vi "Invert_Digital_Data.vi"(8 "error in (no error)":errorcluster, 10 "Index to invert":i32=3, 11 "DO WF":digitalwaveform[](graph)=[{"t0"=timestamp(0 s since 1904-01-01), "dt"=0.0001, "Y"={"transitions"=[], "data"=array90000x1[90000 elements]}}, {"t0"=timestamp(0 s since 1904-01-01), "dt"=0.0001, "Y"={"transitions"=[], "data"=array90000x1[90000 elements]}}, {"t0"=timestamp(0 s since 1904-01-01), "dt"=0.0001, "Y"={"transitions"=[], "data"=array90000x1[90000 elements]}}]) -> (0 "error out":errorcluster, 3 "DO WF 2":digitalwaveform[](graph)=[{"t0"=timestamp(0 s since 1904-01-01), "dt"=0.0001, "Y"={"transitions"=[], "data"=array90000x1[90000 elements]}}, {"t0"=timestamp(0 s since 1904-01-01), "dt"=0.0001, "Y"={"transitions"=[], "data"=array90000x1[90000 elements]}}, {"t0"=timestamp(0 s since 1904-01-01), "dt"=0.0001, "Y"={"transitions"=[], "data"=array90000x1[90000 elements]}}])   [LabVIEW 2025]
uses:
  <vilib>/Waveform/DTblOps.llb/DTbl Invert Digital.vi
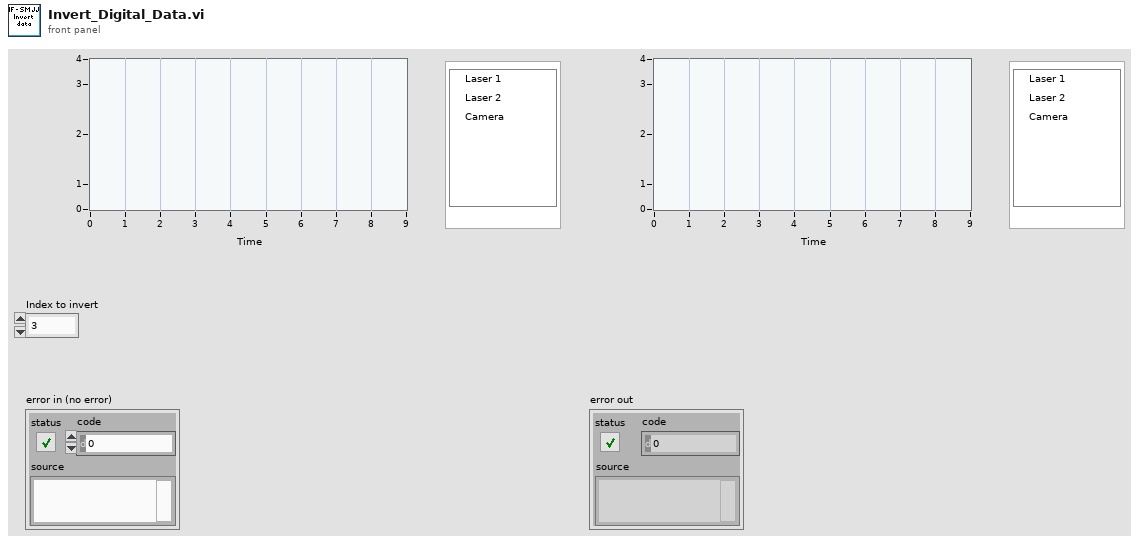
[diagram p1: front panel]
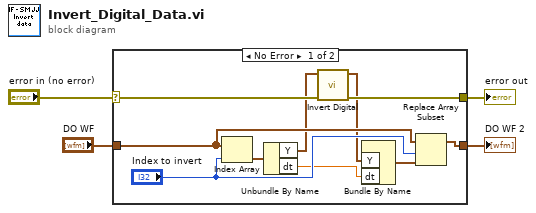
[diagram p0: block diagram]
diagram:
  n1 = case shown="No Error" "error in (no error)" {
    selector: "error in (no error)" -> [w10 w15]
    tunnel: "DO WF" -> [w13 w16]
    tunnel: [w11 w16] -> w3
    tunnel: [w9 w15] -> w1
    frame No Error {
      n2 = Index Array(array=w13, index="Index to invert") -> (element=w14:digitalwaveform)
      n3 = Unbundle By Name(w14) -> ("Y"=w8:digitaldata, "dt"=w6:dbl)
      n4 = call-poly <vilib>:"Invert Digital.vi"("error in (no error)"=w10, "digital data"=w8) -> ("error out"=w9:errorcluster, "inverted digital data"=w7:digitaldata)  [unwired: 8 in]
      n5 = Bundle By Name("Y"=w7, "dt"=w6) -> (w5:digitalwaveform)  [unwired: 1 in]
      n6 = Replace Array Subset(array=w13, new element=w5, index="Index to invert") -> (w11:digitalwaveform[])
    }
    frame Error {
    }
  }
  "DO WF 2" <- w3
  "error out" <- w1
